vi "Get Faults.vi"(6 "Timer(Sec)":dbl=5.0 format="%#_13g", 7 "No of Inputs":i32=5, 11 "Inputs":bool[](array[boolean])) -> (3 "Faults":bool[](array[boolean]))   [LabVIEW 2017]
panel:
  out "x/y":dbl
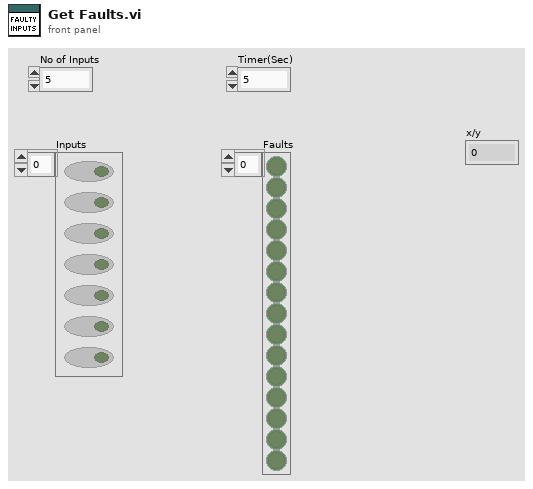
[diagram p1: front panel]
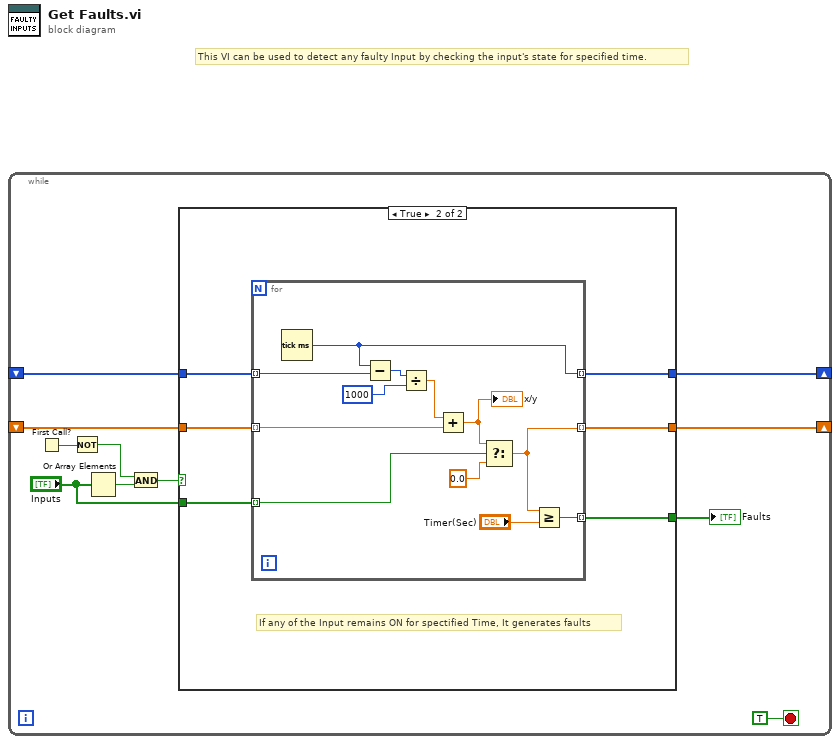
[diagram p0: block diagram]
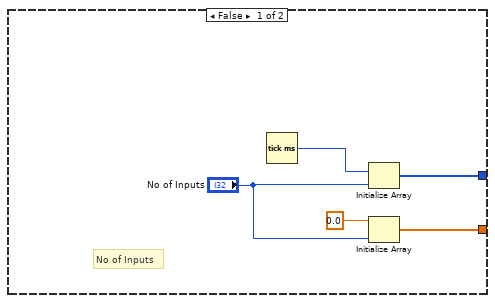
[diagram p2: hidden frame]
diagram:
  # "This VI can be used to detect any faulty Input by checking the input's state for specified time."
  n1 = while {
    shift-right: [w7] -> _
    shift-left: _ -> [w10]
    shift-right: [w5] -> _
    shift-left: _ -> [w4]
    stop <- TRUE ("stop") stop-if-true
    n2 = First Call?() -> (First Call?: T/F=w2:bool)
    n3 = Not(x=w2) -> (.not. x?=w1:bool)
    n4 = Or Array Elements(Boolean array="Inputs") -> (logical OR=w9:bool)
    n5 = And(x=w1, y=w9) -> (x .and. y?=w3:bool)
    n6 = case shown="True" w3 {
      tunnel: w10 -> [_ w22]
      tunnel: "Inputs" -> [_ w20]
      tunnel: [w15 w21] -> w7
      tunnel: [_ w19] -> w6
      tunnel: [w13 w17] -> w5
      tunnel: w4 -> [_ w18]
      frame False {
        # "No of Inputs"
        n7 = Tick Count (ms)() -> (millisecond timer value=w16:u32)
        n8 = Initialize Array(w16, "No of Inputs") -> (w15:u32[])
        n9 = Initialize Array(0.0 ("element"), "No of Inputs") -> (w13:dbl[])
      }
      frame True {
        # "If any of the Input remains ON for spectified Time, It generates faults"
        n10 = for {
          tunnel: w22 -> [w34] mode=indexing
          tunnel: [w27] -> w21 mode=indexing
          tunnel: w20 -> [w31] mode=indexing
          tunnel: [w28] -> w19 mode=indexing
          tunnel: w18 -> [w24] mode=indexing
          tunnel: [w26] -> w17 mode=indexing
          n11 = Tick Count (ms)() -> (millisecond timer value=w27:u32)
          n12 = Subtract(x=w27, y=w34) -> (x-y=w33:u32)
          n13 = Divide(x=w33, y=u32 1000) -> (x/y=w25:dbl)
          n14 = Add(x=w25, y=w24) -> (x+y=w23:dbl)
          "x/y" <- w23
          n15 = Select(t=w23, s=w31, f=0.0) -> (s? t:f=w26:dbl)
          n16 = Greater Or Equal?(x=w26, y="Timer(Sec)") -> (x >= y?=w28:bool)
        }
      }
    }
    "Faults" <- w6
  }
